vi "WritegRPCDetails.vi"(8 "error in (no error)":errorcluster, 10 "gRPCDetails":T1, 11 "MicronGRPCClient in":refnum<class "MicronGRPCClient.lvclass">) -> (0 "error out":errorcluster, 3 "MicronGRPCClient out":refnum<class "MicronGRPCClient.lvclass">)   [LabVIEW 2019, in "MicronGRPCClient.lvclass"]
uses:
  MicronGRPCClient.lvclass
  Typedefs/gRPCDetails.ctl
  <vilib>/gRPC/LabVIEW gRPC Library/Shared/grpcId.ctl
  MicronGRPCClient.lvclass/MicronGRPCClient.ctl
  <vilib>/gRPC/LabVIEW gRPC Library/grpc-lvsupport-release.lvlib
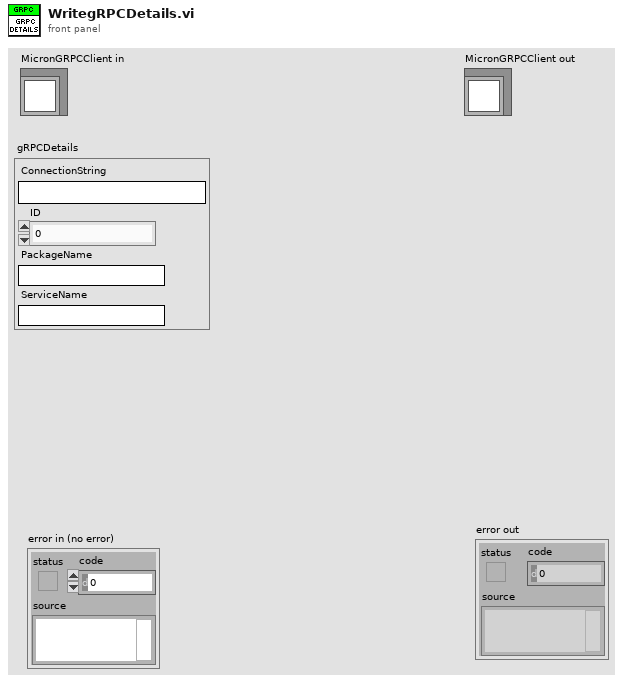
[diagram p1: front panel]
types:
  T1 = typedef "MicronGRPCClient.lvclass/gRPCDetails.ctl" = cluster{"ConnectionString":string, "ID":T2, "PackageName":string, "ServiceName":string}
  T2 = typedef "grpc-lvsupport-release.lvlib/grpcId.ctl" = u64
  T3 = typedef "MicronGRPCClient.lvclass/InternalCluster.ctl" = cluster{"ServiceDetails":T4, "gRPCDetails":T5}
  T4 = typedef "MicronClient.lvclass/ServiceDetails.ctl" = cluster{"MicronPath":path, "Network":string, "ServiceID":string, "Port":i32, "FullyQualifiedName":string, "UI":string, "Args":string, "Mode":string, "AutoRestartOnError?":bool, "Simulate?":bool}
  T5 = typedef "gRPCDetails.ctl" = cluster{"ConnectionString":string, "ID":T2, "PackageName":string, "ServiceName":string}
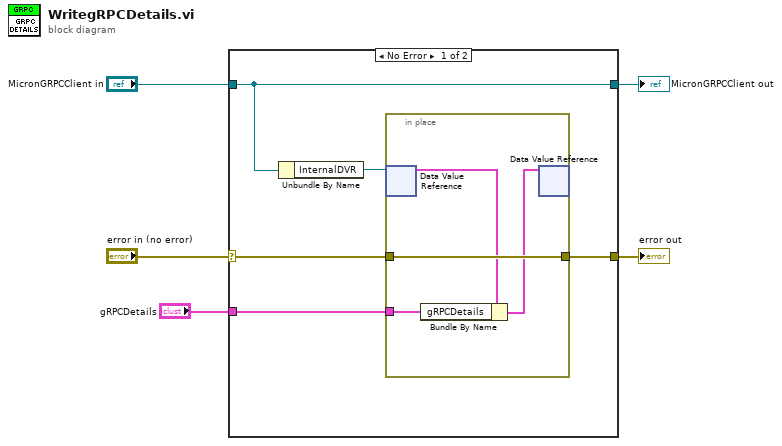
[diagram p0: block diagram]
diagram:
  n1 = case shown="No Error" "error in (no error)" {
    selector: "error in (no error)" -> [w8 w15]
    tunnel: [w7 w15] -> w4
    tunnel: [w10 w16] -> w2
    tunnel: "MicronGRPCClient in" -> [w10 w16]
    tunnel: "gRPCDetails" -> [w6 _]
    frame No Error {
      n2 = Unbundle By Name(w10) -> ("InternalDVR"=w9:refnum<data-value>)
      n3 = in-place {
        in-place-border: w8 -> [w14]
        in-place-border: [w14] -> w7
        in-place-border: w6 -> [w12]
        n4 = in-place-dvr #1(w9) -> (w13:T3)  [unwired: 1 out]
        n5 = Bundle By Name(cluster=w13, "gRPCDetails"=w12) -> (w11:T3)
        n6 = in-place-dvr #1(w11) -> ()  [unwired: 2 out]
      }
    }
    frame Error {
    }
  }
  "error out" <- w4
  "MicronGRPCClient out" <- w2
